vi "main(Test DQMH modules).vi"() -> ()   [LabVIEW 2018, in "Application.lvlib"] (continued)
          frame condition #1 {
          }
        }
        n847 = local read "CE14  Module did it"() -> (w1974:bool[])
        n848 = for {
          N: 6 -> [_]
          tunnel: [w2008] -> w1986 mode=indexing
          tunnel: [w2007] -> w1970 mode=indexing
          i -> [w2010]
          n849 = Increment(x=w2010) -> (x+1=w2009:i32)
          n850 = Wait (ms)(milliseconds to wait=u32 50) -> ()  [unwired: 1 out]
          n851 = call "CE14.CheckConnected.vi"("Module ID"=w2009) -> ("error out"=w2007:errorcluster, "Success"=w2008:bool)  [unwired: 8 in, 1 out]
        }
        "EMIC connected" <- w1986
        n852 = And(x=w1974, y=w1986) -> (x .and. y?=w1977:bool[])
        n853 = Index Array(array=w1977) -> (element #1=→"Inst. 4":bool, element #2=→"Inst. 5":bool, element #3=→"Inst. 6":bool, element #4=→"Inst. 7":bool, element #5=→"Inst. 8":bool, element #6=→"Inst. 9":bool)  [unwired: 6 in]
        n854 = for {
          tunnel: w1977 -> [w1999] mode=indexing
          tunnel: [w1998] -> w1976
          n855 = call "FGV Init phase.vi"("Boolean"=w1999) -> ("Init Completed?"=w1998:bool)  [unwired: 9 in, 1 out]
        }
        n856 = case shown="True" w1976 {
          tunnel: w1975 -> [_ w1997]
          tunnel: [_ w1995] -> w1972
          frame False {
          }
          frame True {
            n857 = call "App enquece.vi"("command"="INIT.Read DRV code", "queue in"=w1997) -> ("error out"=w1995:errorcluster)  [unwired: 8 in, 1 out]
          }
        }
        n858 = Merge Errors(w1971, w1970, w1972) -> (w1973:errorcluster)
        n859 = flat-sequence {
          tunnel: [w2000] -> w1979
          tunnel: w1973 -> [w2000]
          frame #0 {
            n860 = Wait (ms)(milliseconds to wait=u32 70) -> ()  [unwired: 1 out]
          }
        }
      }
      frame "MEAS.Set DMM config" {
        n861 = disable-structure shown="LOGGING==TRUE" {
          disable-tunnel: w2014 -> [w2033 _]
          frame condition #0 (active) {
            n862 = Empty String/Path?(string/path=w2033) -> (empty?=w2035:bool)
            n863 = Select(t="Quece timeout", s=w2035, f=w2033) -> (s? t:f=w2032:string)
            n864 = call "string log (SubVI).vi"("state Name"=w2032) -> ()  [unwired: 9 in, 2 out]
          }
          frame condition #1 {
          }
        }
        n865 = Variant To Data(type=T19 {"DMM config cluster"={"DCV range"=0.0, "DCI range"=0.0, "Detector Rate"=0}, "mux2-1(DMM I) encode"=enum."DMM I (0.5)"} ("DMM all config"), Variant=w2026) -> (data=w2024:T19)  [unwired: 1 in, 1 out]
        n866 = Unbundle By Name(w2024) -> ("DMM config cluster"=w2023:T20)
        n867 = Unbundle By Name(w2023) -> ("DCV range"=w2022:dbl, "DCI range"=w2021:dbl, "Detector Rate"=w2020:u8)
        n868 = call "config channel.vi"("Detector Rate"=w2020, "DCI range"=w2021, "DCV range"=w2022) -> ("error out"=w2018:errorcluster)  [unwired: 8 in]
        n869 = Merge Errors(w2015, w2018) -> (w2012:errorcluster)
        n870 = flat-sequence {
          tunnel: [w2031] -> w2013
          tunnel: w2012 -> [w2031]
          frame #0 {
            n871 = Wait (ms)(milliseconds to wait=u32 70) -> ()  [unwired: 1 out]
          }
        }
      }
      frame "MEAS.AllRelaysOFF" {
        n872 = disable-structure shown="LOGGING==TRUE" {
          disable-tunnel: w2039 -> [w2049 _]
          frame condition #0 (active) {
            n873 = Empty String/Path?(string/path=w2049) -> (empty?=w2051:bool)
            n874 = Select(t="Quece timeout", s=w2051, f=w2049) -> (s? t:f=w2048:string)
            n875 = call "string log (SubVI).vi"("state Name"=w2048) -> ()  [unwired: 9 in, 2 out]
          }
          frame condition #1 {
          }
        }
        n876 = for {
          N: 5 -> [_]
          tunnel: [w2052] -> w2044 mode=indexing
          i -> [w2054]
          n877 = case shown="5.., Default" w2054 {
            tunnel: [w2058 w2059 w2060 w2061 w2062 _] -> w2052
            frame 0 {
              n878 = Initialize Array(FALSE, 6 ("dimension size")) -> (w2055:bool[])
              n879 = call "MB01_eMICs.vi"("Array"=w2055) -> ("error out"=w2058:errorcluster)  [unwired: 10 in]
            }
            frame 1 {
              n880 = call "demux1-10_chan0.vi"() -> ("error out"=w2059:errorcluster)  [unwired: 11 in]
            }
            frame 2 {
              n881 = call "SC enable OFF.vi"() -> ("error out"=w2060:errorcluster)  [unwired: 11 in]
            }
            frame 3 {
              n882 = call "mux10-1_chan0.vi"() -> ("error out"=w2061:errorcluster)  [unwired: 11 in]
            }
            frame 4 {
              n883 = call "mux6-1_chan0.vi"() -> ("error out"=w2062:errorcluster)  [unwired: 11 in]
            }
            frame 5.., Default {
            }
          }
          n884 = Wait (ms)(milliseconds to wait=u32 70) -> ()  [unwired: 1 out]
        }
        n885 = Merge Errors(w2040, w2044) -> (w2037:errorcluster)
      }
      frame "MEAS.AllRelaysOFF2" {
        # "Turn eMICs' relays OFF"
        n886 = disable-structure shown="LOGGING==TRUE" {
          disable-tunnel: w2067 -> [w2080 _]
          frame condition #0 (active) {
            n887 = Empty String/Path?(string/path=w2080) -> (empty?=w2082:bool)
            n888 = Select(t="Quece timeout", s=w2082, f=w2080) -> (s? t:f=w2079:string)
            n889 = call "string log (SubVI).vi"("state Name"=w2079) -> ()  [unwired: 9 in, 2 out]
          }
          frame condition #1 {
          }
        }
        n890 = flat-sequence {
          tunnel: [w2078] -> w2065
          frame #0 {
            n891 = Initialize Array(FALSE, 6 ("dimension size")) -> (w2077:bool[])
            n892 = Wait (ms)(milliseconds to wait=u32 70) -> ()  [unwired: 1 out]
            n893 = call "MB01_eMICs.vi"("Array"=w2077) -> ("error out"=w2078:errorcluster)  [unwired: 10 in]
          }
        }
        n894 = Merge Errors(w2068, w2065) -> (w2064:errorcluster)
      }
      frame "MEAS.Read TRIGGER" {
        w2096 = T8 {"new board?"=TRUE, "new trigger"=TRUE, "last trigger"=TRUE}  # trigger infor
        # "JIG locked - rising-edge event"
        n895 = disable-structure shown="LOGGING==TRUE" {
          disable-tunnel: w2100 -> [w2111 _]
          frame condition #0 (active) {
            n896 = Empty String/Path?(string/path=w2111) -> (empty?=w2113:bool)
            n897 = Select(t="Quece timeout", s=w2113, f=w2111) -> (s? t:f=w2110:string)
            n898 = call "string log (SubVI).vi"("state Name"=w2110) -> ()  [unwired: 9 in, 2 out]
          }
          frame condition #1 {
          }
        }
        n899 = call "Read JIG trigger.vi"() -> ("error out"=w2083:errorcluster, "Trigger?"=w2087:bool)  [unwired: 9 in, 1 out]
        "trigger Value" <- w2087
        n900 = feedback-in #3(w2087) -> ()
        n901 = feedback #3(FALSE) -> (w2094:bool)
        n902 = Greater?(x=w2087, y=w2094) -> (0:w2089:bool)
        n903 = local read "Auto/Man"() -> (w2086:bool)
        n904 = Bundle By Name(cluster=w2096, "new board?"=w2089, "new trigger"=w2087, "last trigger"=w2094) -> (w2095:T8)
        n905 = local write "New board?"(w2089) -> ()
        n906 = local write "new Trigger?"(w2087) -> ()
        n907 = local write "last Trigger?"(w2094) -> ()
        n908 = Select(t=-1, s=w2089, f=w2091) -> (s? t:f=w2092:i32)
        n909 = And(x=w2086, y=w2089) -> (x .and. y?=w2088:bool)
        n910 = case shown="True" w2088 {
          tunnel: w2097 -> [_ w2109]
          tunnel: w2095 -> [_ w2108]
          tunnel: [_ w2107] -> w2084
          frame False {
          }
          frame True {
            n911 = Generate User Event(user event=w2109, event data cluster=w2108) -> (error out=w2107:errorcluster)  [unwired: 2 in, 1 out]
          }
        }
        n912 = Merge Errors(w2085, w2083, w2084) -> (w2098:errorcluster)
        n913 = flat-sequence {
          tunnel: [w2114] -> w2101
          tunnel: w2098 -> [w2114]
          frame #0 {
            n914 = Wait (ms)(milliseconds to wait=u32 10) -> ()  [unwired: 1 out]
          }
        }
      }
      frame "MEAS.Sel Input Current" {
        n915 = disable-structure shown="LOGGING==TRUE" {
          disable-tunnel: w2117 -> [w2132 _]
          frame condition #0 (active) {
            n916 = Empty String/Path?(string/path=w2132) -> (empty?=w2134:bool)
            n917 = Select(t="Quece timeout", s=w2134, f=w2132) -> (s? t:f=w2131:string)
            n918 = call "string log (SubVI).vi"("state Name"=w2131) -> ()  [unwired: 9 in, 2 out]
          }
          frame condition #1 {
          }
        }
        n919 = Variant To Data(type=enum16{"DMM I (0.5)", "DMM I (12)"}."DMM I (0.5)" ("mux2-1(DMM I) encode"), Variant=w2125) -> (data=w2124:enum16{"DMM I (0.5)", "DMM I (12)"})  [unwired: 1 in, 1 out]
        n920 = call "DMM I 0.5_10.vi"("mux2-1(DMM I) encode"=w2124) -> ("error out"=w2127:errorcluster)  [unwired: 10 in]
        n921 = Merge Errors(w2120, w2127) -> (w2118:errorcluster)
        n922 = flat-sequence {
          tunnel: [w2135] -> w2119
          tunnel: w2118 -> [w2135]
          frame #0 {
            n923 = Wait (ms)(milliseconds to wait=u32 70) -> ()  [unwired: 1 out]
          }
        }
      }
      frame "MEAS.Read Optos" {
        n924 = disable-structure shown="LOGGING==TRUE" {
          disable-tunnel: w2141 -> [w2165 _]
          frame condition #0 (active) {
            n925 = Empty String/Path?(string/path=w2165) -> (empty?=w2167:bool)
            n926 = Select(t="Quece timeout", s=w2167, f=w2165) -> (s? t:f=w2164:string)
            n927 = call "string log (SubVI).vi"("state Name"=w2164) -> ()  [unwired: 9 in, 2 out]
          }
          frame condition #1 {
          }
        }
        n928 = flat-sequence {
          tunnel: [w2154] -> w2139
          frame #0 {
            n929 = disable-structure shown="Enabled" {
              frame Enabled {
                n930 = Wait (ms)(milliseconds to wait=u32 100) -> ()  [unwired: 1 out]
              }
              frame Disabled {
              }
            }
            n931 = Initialize Array(FALSE, 6 ("dimension size"), 10 ("dimension size")) -> (w2149:bool[][])
            n932 = local write "Short DRV"(w2149) -> ()
          }
          frame #1 {
            n933 = call "inst.Optos.vi"() -> ("error out"=w2163:errorcluster, "Optos"=w2161:bool[])  [unwired: 9 in, 1 out]
            n934 = Reshape Array(w2161, 10 ("dimension size"), 6 ("dimension size")) -> (w2159:bool[][])
            n935 = To Variant(anything=w2161) -> (Variant=w2162:variant)
            n936 = Transpose 2D Array(2D array=w2159) -> (transposed array=→"Short DRV":bool[][])
            n937 = call "FGV Driver Data.vi"("Mode"=DUT_data_Mode."Short Circuits", "error in (no error)"=w2163, "FGV enum(Read)"=FGV_DRV_data."Write" ("FGV DRV data enum"), "data"=w2162) -> ("error out"=w2154:errorcluster)  [unwired: 4 in, 3 out]
          }
        }
        n938 = Merge Errors(w2140, w2139) -> (w2137:errorcluster)
        n939 = flat-sequence {
          tunnel: [w2168] -> w2142
          tunnel: w2137 -> [w2168]
          frame #0 {
            n940 = Wait (ms)(milliseconds to wait=u32 70) -> ()  [unwired: 1 out]
          }
        }
      }
      frame "MEAS.Reset JIG" {
        n941 = disable-structure shown="LOGGING==TRUE" {
          disable-tunnel: w2174 -> [w2185 _]
          frame condition #0 (active) {
            n942 = Empty String/Path?(string/path=w2185) -> (empty?=w2187:bool)
            n943 = Select(t="Quece timeout", s=w2187, f=w2185) -> (s? t:f=w2184:string)
            n944 = call "string log (SubVI).vi"("state Name"=w2184) -> ()  [unwired: 9 in, 2 out]
          }
          frame condition #1 {
          }
        }
        n945 = call "JIG Reset.vi"() -> ("error out"=w2179:errorcluster)  [unwired: 11 in]
        n946 = Merge Errors(w2175, w2179) -> (w2170:errorcluster)
        n947 = flat-sequence {
          tunnel: [w2182] -> w2171
          tunnel: w2170 -> [w2182]
          frame #0 {
            n948 = Wait (ms)(milliseconds to wait=u32 100) -> ()  [unwired: 1 out]
          }
        }
      }
      frame "MEAS.Turn+5V" {
        n949 = disable-structure shown="LOGGING==TRUE" {
          disable-tunnel: w2190 -> [w2206 _]
          frame condition #0 (active) {
            n950 = Empty String/Path?(string/path=w2206) -> (empty?=w2208:bool)
            n951 = Select(t="Quece timeout", s=w2208, f=w2206) -> (s? t:f=w2205:string)
            n952 = call "string log (SubVI).vi"("state Name"=w2205) -> ()  [unwired: 9 in, 2 out]
          }
          frame condition #1 {
          }
        }
        n953 = Variant To Data(type=TRUE, Variant=w2199) -> (data=w2189:bool)  [unwired: 1 in, 1 out]
        n954 = case shown="False" w2189 {
          tunnel: [w2203 w2204] -> w2196
          frame False {
            n955 = call "SC enable OFF.vi"() -> ("error out"=w2203:errorcluster)  [unwired: 11 in]
          }
          frame True {
            n956 = call "SC enable ON.vi"() -> ("error out"=w2204:errorcluster)  [unwired: 11 in]
          }
        }
        n957 = Merge Errors(w2191, w2196) -> (w2192:errorcluster)
        n958 = flat-sequence {
          tunnel: w2192 -> [w2209]
          tunnel: [w2209] -> w2195
          frame #0 {
            n959 = Wait (ms)(milliseconds to wait=u32 2000) -> ()  [unwired: 1 out]
          }
        }
      }
      frame "MEAS.demux1-10" {
        n960 = disable-structure shown="LOGGING==TRUE" {
          disable-tunnel: w2214 -> [w2240 _]
          frame condition #0 (active) {
            n961 = Empty String/Path?(string/path=w2240) -> (empty?=w2242:bool)
            n962 = Select(t="Quece timeout", s=w2242, f=w2240) -> (s? t:f=w2239:string)
            n963 = call "string log (SubVI).vi"("state Name"=w2239) -> ()  [unwired: 9 in, 2 out]
          }
          frame condition #1 {
          }
        }
        n964 = Variant To Data(type=T4."demux1_10_channel0" ("demux1_10(x6)_encode"), Variant=w2222) -> (data=w2213:T4)  [unwired: 1 in, 1 out]
        n965 = case shown="\"demux1_10_channel7\"" w2213 {
          tunnel: [w2228 w2229 w2230 w2231 w2232 w2233 w2234 w2235 w2236 w2237 w2238] -> w2212
          frame "demux1_10_channel0", Default {
            n966 = call "demux1-10_chan0.vi"() -> ("error out"=w2228:errorcluster)  [unwired: 11 in]
          }
          frame "demux1_10_channel1" {
            n967 = call "demux1-10_chan1.vi"() -> ("error out"=w2229:errorcluster)  [unwired: 11 in]
          }
          frame "demux1_10_channel2" {
            n968 = call "demux1-10_chan2.vi"() -> ("error out"=w2230:errorcluster)  [unwired: 11 in]
          }
          frame "demux1_10_channel3" {
            n969 = call "demux1-10_chan3.vi"() -> ("error out"=w2231:errorcluster)  [unwired: 11 in]
          }
          frame "demux1_10_channel4" {
            n970 = call "demux1-10_chan4.vi"() -> ("error out"=w2232:errorcluster)  [unwired: 11 in]
          }
          frame "demux1_10_channel5" {
            n971 = call "demux1-10_chan5.vi"() -> ("error out"=w2233:errorcluster)  [unwired: 11 in]
          }
          frame "demux1_10_channel6" {
            n972 = call "demux1-10_chan6.vi"() -> ("error out"=w2234:errorcluster)  [unwired: 11 in]
          }
          frame "demux1_10_channel7" {
            n973 = call "demux1-10_chan7.vi"() -> ("error out"=w2235:errorcluster)  [unwired: 11 in]
          }
          frame "demux1_10_channel8" {
            n974 = call "demux1-10_chan8.vi"() -> ("error out"=w2236:errorcluster)  [unwired: 11 in]
          }
          frame "demux1_10_channel9" {
            n975 = call "demux1-10_chan9.vi"() -> ("error out"=w2237:errorcluster)  [unwired: 11 in]
          }
          frame "demux1_10_channel10" {
            n976 = call "demux1-10_chan10.vi"() -> ("error out"=w2238:errorcluster)  [unwired: 11 in]
          }
        }
        n977 = Merge Errors(w2215, w2212) -> (w2216:errorcluster)
        n978 = flat-sequence {
          tunnel: [w2226] -> w2217
          tunnel: w2216 -> [w2226]
          frame #0 {
            n979 = Wait (ms)(milliseconds to wait=u32 100 ("1-10delay")) -> ()  [unwired: 1 out]
          }
        }
      }
      frame "MEAS.eMIC" {
        # "eliminated shorted Circuits"
        n980 = disable-structure shown="LOGGING==TRUE" {
          disable-tunnel: w2245 -> [w2267 _]
          frame condition #0 (active) {
            n981 = Empty String/Path?(string/path=w2267) -> (empty?=w2269:bool)
            n982 = Select(t="Quece timeout", s=w2269, f=w2267) -> (s? t:f=w2266:string)
            n983 = call "string log (SubVI).vi"("state Name"=w2266) -> ()  [unwired: 9 in, 2 out]
          }
          frame condition #1 {
          }
        }
        n984 = Variant To Data(type=bool[] [], Variant=w2260) -> (data=w2254:bool[])  [unwired: 1 in, 1 out]
        n985 = call "FGV Driver Data.vi"("DUT channel (1-11)"=w2247) -> ("Short Circuits?"=w2256:bool[])  [unwired: 7 in, 3 out]
        n986 = Not(x=w2256) -> (.not. x?=w2255:bool[])
        n987 = And(x=w2255, y=w2254) -> (x .and. y?=w2253:bool[])
        n988 = call "MB01_eMICs.vi"("Array"=w2253) -> ("error out"=w2251:errorcluster)  [unwired: 10 in]
        n989 = call "FGV wait for 6 eMICs.vi"("Enum"=enum16{"Init", "count"}."Init", "error in (no error)"=w2251) -> ("error out"=w2243:errorcluster, "wait done"=w2252:bool)  [unwired: 7 in, 1 out]
        n990 = local write "AC  Completed"(w2252) -> ()
        n991 = Merge Errors(w2246, w2243) -> (w2248:errorcluster)
        n992 = flat-sequence {
          tunnel: [w2265] -> w2249
          tunnel: w2248 -> [w2265]
          frame #0 {
            n993 = Wait (ms)(milliseconds to wait=u32 100 ("eMIC delay")) -> ()  [unwired: 1 out]
          }
        }
      }
      frame "MEAS.requestAC" {
        n994 = disable-structure shown="LOGGING==TRUE" {
          disable-tunnel: w2273 -> [w2296 _]
          frame condition #0 (active) {
            n995 = Empty String/Path?(string/path=w2296) -> (empty?=w2298:bool)
            n996 = Select(t="Quece timeout", s=w2298, f=w2296) -> (s? t:f=w2295:string)
            n997 = call "string log (SubVI).vi"("state Name"=w2295) -> ()  [unwired: 9 in, 2 out]
          }
          frame condition #1 {
          }
        }
        n998 = Variant To Data(type=-1 ("Module ID"), Variant=w2271) -> (data=w2270:i32)  [unwired: 1 in, 1 out]
        n999 = case shown="1, Default" w2270 {
          selector: w2270 -> [w2289 _]
          tunnel: [w2288 w2293] -> w2276
          frame 1, Default {
            n1000 = Quotient & Remainder(x=w2289, y=6) -> (x-y*floor(x/y)=w2285:i32)  [unwired: 1 out]
            n1001 = Equal To 0?(x=w2285) -> (x = 0?=w2287:bool)
            n1002 = Select(t=6, s=w2287, f=w2285) -> (s? t:f=w2284:i32)
            n1003 = call "Read AC parameters.vi"("Module ID"=w2284) -> ("error out"=w2288:errorcluster)  [unwired: 10 in]
          }
          frame 0 {
            n1004 = call "FGV wait for 6 eMICs.vi"("Enum"=enum16{"Init", "count"}."Init") -> ("error out"=w2291:errorcluster)  [unwired: 8 in, 2 out]
            n1005 = call "Read AC parameters.vi"("error in"=w2291, "Module ID"=-1) -> ("error out"=w2293:errorcluster)  [unwired: 9 in]
          }
        }
        n1006 = Merge Errors(w2277, w2276) -> (w2275:errorcluster)
      }
      frame "MEAS.mux6_1" {
        n1007 = disable-structure shown="LOGGING==TRUE" {
          disable-tunnel: w2306 -> [w2343 _]
          frame condition #0 (active) {
            n1008 = Empty String/Path?(string/path=w2343) -> (empty?=w2345:bool)
            n1009 = Select(t="Quece timeout", s=w2345, f=w2343) -> (s? t:f=w2342:string)
            n1010 = call "string log (SubVI).vi"("state Name"=w2342) -> ()  [unwired: 9 in, 2 out]
          }
          frame condition #1 {
          }
        }
        n1011 = Variant To Data(type=T2."mux6-1_channel0" ("mux6_1(3wires)_encode"), Variant=w2312) -> (data=w2305:T2)  [unwired: 1 in, 1 out]
        n1012 = case shown="\"mux6_1_channel1_3\"" w2305 {
          tunnel: [w2317 w2319 w2321 w2323 w2325 w2327 w2329 w2331 w2333 w2335 w2337 w2339 w2341] -> w2304
          tunnel: [w2316 w2318 w2320 w2322 w2324 w2326 w2328 w2330 w2332 w2334 w2336 w2338 w2340] -> w2300
          tunnel: u32 180 ("6_1 delay") -> [w2316 _ w2320 _ w2324 _ w2328 _ w2332 _ w2336 _ w2340]
          tunnel: u32 70 ("6_1 delay2") -> [_ w2318 _ w2322 _ w2326 _ w2330 _ w2334 _ w2338 _]
          frame "mux6-1_channel0", Default {
            n1013 = call "mux6-1_chan0.vi"() -> ("error out"=w2317:errorcluster)  [unwired: 11 in]
          }
          frame "mux6-1_channel1_2" {
            n1014 = call "mux6-1_chan1_1.vi"() -> ("error out"=w2319:errorcluster)  [unwired: 11 in]
          }
          frame "mux6_1_channel1_3" {
            n1015 = call "mux6-1_chan1_2.vi"() -> ("error out"=w2321:errorcluster)  [unwired: 11 in]
          }
          frame "mux6_1_channel2_2" {
            n1016 = call "mux6-1_chan2_1.vi"() -> ("error out"=w2323:errorcluster)  [unwired: 11 in]
          }
          frame "mux6_1_channel2_3" {
            n1017 = call "mux6-1_chan2_2.vi"() -> ("error out"=w2325:errorcluster)  [unwired: 11 in]
          }
          frame "mux6_1_channel3_2" {
            n1018 = call "mux6-1_chan3_1.vi"() -> ("error out"=w2327:errorcluster)  [unwired: 11 in]
          }
          frame "mux6_1_channel3_3" {
            n1019 = call "mux6-1_chan3_2.vi"() -> ("error out"=w2329:errorcluster)  [unwired: 11 in]
          }
          frame "mux6_1_channel4_2" {
            n1020 = call "mux6-1_chan4_1.vi"() -> ("error out"=w2331:errorcluster)  [unwired: 11 in]
          }
          frame "mux6_1_channel4_3" {
            n1021 = call "mux6-1_chan4_2.vi"() -> ("error out"=w2333:errorcluster)  [unwired: 11 in]
          }
          frame "mux6_1_channel5_2" {
            n1022 = call "mux6-1_chan5_1.vi"() -> ("error out"=w2335:errorcluster)  [unwired: 11 in]
          }
          frame "mux6_1_channel5_3" {
            n1023 = call "mux6-1_chan5_2.vi"() -> ("error out"=w2337:errorcluster)  [unwired: 11 in]
          }
          frame "mux6_1_channel6_2" {
            n1024 = call "mux6-1_chan6_1.vi"() -> ("error out"=w2339:errorcluster)  [unwired: 11 in]
          }
          frame "mux6_1_channel6_3" {
            n1025 = call "mux6-1_chan6_2.vi"() -> ("error out"=w2341:errorcluster)  [unwired: 11 in]
          }
        }
        n1026 = Wait (ms)(milliseconds to wait=w2300) -> ()  [unwired: 1 out]
        n1027 = Merge Errors(w2307, w2304) -> (w2299:errorcluster)
      }
      frame "MEAS.mux10-1" {
        n1028 = disable-structure shown="LOGGING==TRUE" {
          disable-tunnel: w2349 -> [w2375 _]
          frame condition #0 (active) {
            n1029 = Empty String/Path?(string/path=w2375) -> (empty?=w2377:bool)
            n1030 = Select(t="Quece timeout", s=w2377, f=w2375) -> (s? t:f=w2374:string)
            n1031 = call "string log (SubVI).vi"("state Name"=w2374) -> ()  [unwired: 9 in, 2 out]
          }
          frame condition #1 {
          }
        }
        n1032 = Variant To Data(type=T3."mux10_1_channel0" ("mux10_1(x6)_encode"), Variant=w2357) -> (data=w2348:T3)  [unwired: 1 in, 1 out]
        n1033 = case shown="\"mux10_1_channel10\"" w2348 {
          tunnel: [w2363 w2364 w2365 w2366 w2367 w2368 w2369 w2370 w2371 w2372 w2373] -> w2347
          frame "mux10_1_channel0", Default {
            n1034 = call "mux10-1_chan0.vi"() -> ("error out"=w2363:errorcluster)  [unwired: 11 in]
          }
          frame "mux10_1_channel1" {
            n1035 = call "mux10-1_chan1.vi"() -> ("error out"=w2364:errorcluster)  [unwired: 11 in]
          }
          frame "mux10_1_channel2" {
            n1036 = call "mux10-1_chan2.vi"() -> ("error out"=w2365:errorcluster)  [unwired: 11 in]
          }
          frame "mux10_1_channel3" {
            n1037 = call "mux10-1_chan3.vi"() -> ("error out"=w2366:errorcluster)  [unwired: 11 in]
          }
          frame "mux10_1_channel4" {
            n1038 = call "mux10-1_chan4.vi"() -> ("error out"=w2367:errorcluster)  [unwired: 11 in]
          }
          frame "mux10_1_channel5" {
            n1039 = call "mux10-1_chan5.vi"() -> ("error out"=w2368:errorcluster)  [unwired: 11 in]
          }
          frame "mux10_1_channel6" {
            n1040 = call "mux10-1_chan6.vi"() -> ("error out"=w2369:errorcluster)  [unwired: 11 in]
          }
          frame "mux10_1_channel7" {
            n1041 = call "mux10-1_chan7.vi"() -> ("error out"=w2370:errorcluster)  [unwired: 11 in]
          }
          frame "mux10_1_channel8" {
            n1042 = call "mux10-1_chan8.vi"() -> ("error out"=w2371:errorcluster)  [unwired: 11 in]
          }
          frame "mux10_1_channel9" {
            n1043 = call "mux10-1_chan9.vi"() -> ("error out"=w2372:errorcluster)  [unwired: 11 in]
          }
          frame "mux10_1_channel10" {
            n1044 = call "mux10-1_chan10.vi"() -> ("error out"=w2373:errorcluster)  [unwired: 11 in]
          }
        }
        n1045 = Merge Errors(w2352, w2347) -> (w2351:errorcluster)
        n1046 = flat-sequence {
          tunnel: w2351 -> [w2361]
          tunnel: [w2361] -> w2350
          frame #0 {
            n1047 = Wait (ms)(milliseconds to wait=u32 100 ("10-1 delay")) -> ()  [unwired: 1 out]
          }
        }
      }
      frame "MEAS.DMM dual read" {
        n1048 = disable-structure shown="LOGGING==TRUE" {
          disable-tunnel: w2385 -> [w2410 _]
          frame condition #0 (active) {
            n1049 = Empty String/Path?(string/path=w2410) -> (empty?=w2413:bool)
            n1050 = Select(t="Quece timeout", s=w2413, f=w2410) -> (s? t:f=w2411:string)
            n1051 = call "string log (SubVI).vi"("state Name"=w2411) -> ()  [unwired: 9 in, 2 out]
          }
          frame condition #1 {
          }
        }
        n1052 = call "FGV Driver Data.vi"("DUT index(1-60)"=w2378) -> ("DUT SC"=w2379:bool)  [unwired: 7 in, 3 out]
        n1053 = case shown="True" w2379 {
          tunnel: [w2392 _] -> w2381
          tunnel: w2378 -> [w2393 _]
          frame False {
            n1054 = flat-sequence {
              tunnel: [w2396] -> w2394
              tunnel: w2393 -> [w2396]
              tunnel: w2394 -> [w2399]
              tunnel: [w2398] -> w2392
              frame #0 {
                w2395 = 0.0 ("DCV(Volts)")
                n1055 = disable-structure shown="Enabled" {
                  frame Enabled {
                    n1056 = Wait (ms)(milliseconds to wait=u32 50) -> ()  [unwired: 1 out]
                  }
                  frame Disabled {
                  }
                }
                n1057 = local write "DCV(Volts)"(w2395) -> ()
                n1058 = local write "DCI(mA)"(w2395) -> ()
              }
              frame #1 {
                w2400 = u16 2 items=["1st Display", "2nd Display", "1st & 2nd Display"] ("Sets to Display")
                n1059 = call "Read DCV_DCI.vi"("Sets to Display"=w2400) -> ("error out"=w2403:errorcluster, "DCI"=w2407:dbl, "DCV"=w2406:dbl)  [unwired: 7 in, 1 out]
                "DCI(mA)" <- w2407
                "DCV(Volts)" <- w2406
                n1060 = Build Array(w2406, w2407) -> (w2405:dbl[])
                n1061 = To Variant(anything=w2405) -> (Variant=w2404:variant)
                n1062 = call "FGV Driver Data.vi"("Mode"=DUT_data_Mode."DC parameter", "DUT index(1-60)"=w2399, "error in (no error)"=w2403, "FGV enum(Read)"=FGV_DRV_data."Write" ("FGV DRV data enum"), "data"=w2404) -> ("error out"=w2398:errorcluster)  [unwired: 3 in, 3 out]
              }
            }
          }
          frame True {
          }
        }
        n1063 = Merge Errors(w2386, w2381) -> (w2383:errorcluster)
        n1064 = flat-sequence {
          tunnel: [w2409] -> w2384
          tunnel: w2383 -> [w2409]
          frame #0 {
            n1065 = Wait (ms)(milliseconds to wait=u32 10 ("DMM delay")) -> ()  [unwired: 1 out]
          }
        }
      }
      frame "Test Shorted Circuits" {
        w2422 = T24 {"command"="", "Data"=variant} ("Variant")
        n1066 = disable-structure shown="LOGGING==TRUE" {
          disable-tunnel: w2428 -> [w2448 _]
          frame condition #0 (active) {
            n1067 = Empty String/Path?(string/path=w2448) -> (empty?=w2450:bool)
            n1068 = Select(t="Quece timeout", s=w2450, f=w2448) -> (s? t:f=w2447:string)
            n1069 = call "string log (SubVI).vi"("state Name"=w2447) -> ()  [unwired: 9 in, 2 out]
          }
          frame condition #1 {
          }
        }
        n1070 = To Variant(anything=TRUE) -> (Variant=w2438:variant)
        n1071 = To Variant(anything=FALSE) -> (Variant=w2424:variant)
        n1072 = Bundle By Name(cluster=w2422, "command"="MEAS.AllRelaysOFF") -> (w2440:T24)
        n1073 = Bundle By Name(cluster=w2422, "command"="MEAS.Turn+5V", "Data"=w2438) -> (w2439:T24)
        n1074 = Bundle By Name(cluster=w2422, "command"="MEAS.Read Optos") -> (w2436:T24)
        n1075 = Bundle By Name(cluster=w2422, "command"="MEAS.Turn+5V", "Data"=w2424) -> (w2427:T24)
        n1076 = Bundle By Name(cluster=w2422, "command"="Apps.UI Update SC") -> (w2420:T24)
        n1077 = Build Array(w2440, w2439, w2436, w2427, w2420) -> (w2429:T24[])
        n1078 = Reverse 1D Array(array=w2429) -> (reversed array=w2430:T24[])
        n1079 = for {
          tunnel: w2430 -> [w2454] mode=indexing
          tunnel: w2434 -> [w2456]
          tunnel: [w2455] -> w2414 mode=indexing
          n1080 = Unbundle By Name(w2454) -> ("command"=w2453:string, "Data"=w2452:variant)
          n1081 = call "App enquece.vi"("Priority Enquece"=TRUE, "command data"=w2452, "command"=w2453, "queue in"=w2456) -> ("error out"=w2455:errorcluster)  [unwired: 6 in, 1 out]
        }
        n1082 = call "reset DRV UI (SubVI).vi"("Ref  in"=w2433) -> ("error out"=w2417:errorcluster)  [unwired: 9 in, 1 out]
        n1083 = call "FGV Driver Data.vi"("error in (no error)"=w2417, "FGV enum(Read)"=FGV_DRV_data."Init" ("FGV DRV data enum")) -> ("error out"=w2415:errorcluster)  [unwired: 6 in, 3 out]
        n1084 = Merge Errors(w2416, w2415, w2414) -> (w2419:errorcluster)
      }
      frame "Test Channel 1" {
        w2463 = T9 {"command"="", "data"=variant} ("element")
        w2497 = 1  # DUT channel (1-11)
        n1085 = disable-structure shown="LOGGING==TRUE" {
          disable-tunnel: w2493 -> [w2523 _]
          frame condition #0 (active) {
            n1086 = Empty String/Path?(string/path=w2523) -> (empty?=w2525:bool)
            n1087 = Select(t="Quece timeout", s=w2525, f=w2523) -> (s? t:f=w2522:string)
            n1088 = call "string log (SubVI).vi"("state Name"=w2522) -> ()  [unwired: 9 in, 2 out]
          }
          frame condition #1 {
          }
        }
        n1089 = Build Array("Apps.WaitForEvent", "MEAS.AllRelaysOFF2", "Apps.UI Update") -> (w2459:string[])
        n1090 = Reverse 1D Array(array=w2459) -> (reversed array=w2458:string[])
        n1091 = for {
          tunnel: [w2513] -> w2483 mode=indexing
          shift-right: [w2512] -> w2482
          shift-left: w2484 -> [w2515]
          tunnel: w2458 -> [w2511] mode=indexing
          n1092 = call "App enquece.vi"("Priority Enquece"=TRUE, "command"=w2511, "queue in"=w2515) -> ("error out"=w2513:errorcluster, "Queue out"=w2512:refnum<queue>)  [unwired: 7 in]
        }
        n1093 = call "FGV DRV stand.vi"() -> ("Sub-Test.DCV"=w2477:bool)  [unwired: 10 in, 1 out]
        n1094 = Merge Errors(w2483) -> (w2480:errorcluster)
        n1095 = case shown="False" w2477 {
          tunnel: [w2500 w2510] -> w2490
          frame False {
            n1096 = Build Array("WaitFor", "MEAS.requestAC") -> (w2500:string[])
          }
          frame True {
            n1097 = Build Array("Test DRV 1", "Test DRV 2", "Test DRV 3", "Test DRV 4", "Test DRV 5", "Test DRV 6", "MEAS.requestAC") -> (w2510:string[])
          }
        }
        n1098 = Reverse 1D Array(array=w2490) -> (reversed array=w2491:string[])
        n1099 = for {
          tunnel: w2491 -> [w2520] mode=indexing
          tunnel: [w2519] -> w2488 mode=indexing
          shift-right: [w2518] -> w2489
          shift-left: w2482 -> [w2521]
          tunnel: w2480 -> [w2517]
          n1100 = call "App enquece.vi"("Priority Enquece"=TRUE, "error in (no error)"=w2517, "command"=w2520, "queue in"=w2521) -> ("error out"=w2519:errorcluster, "Queue out"=w2518:refnum<queue>)  [unwired: 6 in]
        }
        n1101 = Merge Errors(w2488) -> (w2487:errorcluster)
        n1102 = Initialize Array(TRUE, 6 ("dimension size")) -> (w2465:bool[])
        n1103 = To Variant(anything=T3."mux10_1_channel1" ("mux10_1(x6)_encode")) -> (Variant=w2475:variant)
        n1104 = To Variant(anything=T4."demux1_10_channel1" ("demux1_10(x6)_encode")) -> (Variant=w2471:variant)
        n1105 = To Variant(anything=w2465) -> (Variant=w2464:variant)
        n1106 = Bundle By Name(cluster=w2463, "command"="MEAS.mux10-1", "data"=w2475) -> (w2470:T9)
        n1107 = Bundle By Name(cluster=w2463, "command"="MEAS.demux1-10", "data"=w2471) -> (w2469:T9)
        n1108 = Bundle By Name(cluster=w2463, "command"="MEAS.eMIC", "data"=w2464) -> (w2457:T9)
        n1109 = Build Array(w2470, w2469, w2457, w2457) -> (w2486:T9[])
        n1110 = Reverse 1D Array(array=w2486) -> (reversed array=w2485:T9[])
        n1111 = for {
          tunnel: w2485 -> [w2531] mode=indexing
          tunnel: [w2528] -> w2492 mode=indexing
          tunnel: w2487 -> [w2527]
          tunnel: w2489 -> [w2532]
          n1112 = Unbundle By Name(w2531) -> ("command"=w2530:string, "data"=w2529:variant)
          n1113 = call "App enquece.vi"("Priority Enquece"=TRUE, "error in (no error)"=w2527, "command data"=w2529, "command"=w2530, "queue in"=w2532) -> ("error out"=w2528:errorcluster)  [unwired: 5 in, 1 out]
        }
        n1114 = Merge Errors(w2495, w2492) -> (w2496:errorcluster)
      }
      frame "Test Channel 2" {
        w2539 = T9 {"command"="", "data"=variant} ("element")
        w2573 = 2  # DUT channel (1-11)
        n1115 = disable-structure shown="LOGGING==TRUE" {
          disable-tunnel: w2568 -> [w2599 _]
          frame condition #0 (active) {
            n1116 = Empty String/Path?(string/path=w2599) -> (empty?=w2601:bool)
            n1117 = Select(t="Quece timeout", s=w2601, f=w2599) -> (s? t:f=w2598:string)
            n1118 = call "string log (SubVI).vi"("state Name"=w2598) -> ()  [unwired: 9 in, 2 out]
          }
          frame condition #1 {
          }
        }
        n1119 = Build Array("Apps.WaitForEvent", "MEAS.AllRelaysOFF2", "Apps.UI Update") -> (w2536:string[])
        n1120 = Reverse 1D Array(array=w2536) -> (reversed array=w2535:string[])
        n1121 = for {
          tunnel: [w2590] -> w2562 mode=indexing
          shift-right: [w2591] -> w2564
          shift-left: w2557 -> [w2589]
          tunnel: w2535 -> [w2587] mode=indexing
          n1122 = call "App enquece.vi"("Priority Enquece"=TRUE, "command"=w2587, "queue in"=w2589) -> ("error out"=w2590:errorcluster, "Queue out"=w2591:refnum<queue>)  [unwired: 7 in]
        }
        n1123 = call "FGV DRV stand.vi"() -> ("Sub-Test.DCV"=w2552:bool)  [unwired: 10 in, 1 out]
        n1124 = case shown="True" w2552 {
          tunnel: [w2576 w2586] -> w2565
          frame False {
            n1125 = Build Array("WaitFor", "MEAS.requestAC") -> (w2576:string[])
          }
          frame True {
            n1126 = Build Array("Test DRV 7", "Test DRV 8", "Test DRV 9", "Test DRV 10", "Test DRV 11", "Test DRV 12", "MEAS.requestAC") -> (w2586:string[])
          }
        }
        n1127 = Merge Errors(w2562) -> (w2556:errorcluster)
        n1128 = Reverse 1D Array(array=w2565) -> (reversed array=w2566:string[])
        n1129 = for {
          tunnel: w2566 -> [w2592] mode=indexing
          tunnel: [w2596] -> w2561 mode=indexing
          shift-right: [w2595] -> w2563
          shift-left: w2564 -> [w2597]
          tunnel: w2556 -> [w2594]
          n1130 = call "App enquece.vi"("Priority Enquece"=TRUE, "error in (no error)"=w2594, "command"=w2592, "queue in"=w2597) -> ("error out"=w2596:errorcluster, "Queue out"=w2595:refnum<queue>)  [unwired: 6 in]
        }
        n1131 = Merge Errors(w2561) -> (w2560:errorcluster)
        n1132 = Initialize Array(TRUE, 6 ("dimension size")) -> (w2542:bool[])
        n1133 = To Variant(anything=T3."mux10_1_channel2" ("mux10_1(x6)_encode")) -> (Variant=w2550:variant)
        n1134 = To Variant(anything=T4."demux1_10_channel2" ("demux1_10(x6)_encode")) -> (Variant=w2547:variant)
        n1135 = To Variant(anything=w2542) -> (Variant=w2541:variant)
        n1136 = Bundle By Name(cluster=w2539, "command"="MEAS.mux10-1", "data"=w2550) -> (w2546:T9)
        n1137 = Bundle By Name(cluster=w2539, "command"="MEAS.demux1-10", "data"=w2547) -> (w2545:T9)
        n1138 = Bundle By Name(cluster=w2539, "command"="MEAS.eMIC", "data"=w2541) -> (w2540:T9)
        n1139 = Build Array(w2546, w2545, w2540) -> (w2559:T9[])
        n1140 = Reverse 1D Array(array=w2559) -> (reversed array=w2558:T9[])
        n1141 = for {
          tunnel: w2558 -> [w2607] mode=indexing
          tunnel: [w2604] -> w2567 mode=indexing
          tunnel: w2560 -> [w2603]
          tunnel: w2563 -> [w2608]
          n1142 = Unbundle By Name(w2607) -> ("command"=w2606:string, "data"=w2605:variant)
          n1143 = call "App enquece.vi"("Priority Enquece"=TRUE, "error in (no error)"=w2603, "command data"=w2605, "command"=w2606, "queue in"=w2608) -> ("error out"=w2604:errorcluster)  [unwired: 5 in, 1 out]
        }
        n1144 = Merge Errors(w2570, w2567) -> (w2571:errorcluster)
      }
      frame "Test Channel 3" {
        w2612 = T9 {"command"="", "data"=variant} ("element")
        w2648 = 3  # DUT channel (1-11)
        n1145 = disable-structure shown="LOGGING==TRUE" {
          disable-tunnel: w2644 -> [w2674 _]
          frame condition #0 (active) {
            n1146 = Empty String/Path?(string/path=w2674) -> (empty?=w2676:bool)
            n1147 = Select(t="Quece timeout", s=w2676, f=w2674) -> (s? t:f=w2673:string)
            n1148 = call "string log (SubVI).vi"("state Name"=w2673) -> ()  [unwired: 9 in, 2 out]
          }
          frame condition #1 {
          }
        }
        n1149 = Build Array("Apps.UI Update", "MEAS.AllRelaysOFF2", "Apps.WaitForEvent") -> (w2632:string[])
        n1150 = for {
          tunnel: [w2664] -> w2638 mode=indexing
          shift-right: [w2665] -> w2640
          shift-left: w2634 -> [w2663]
          tunnel: w2632 -> [w2662] mode=indexing
          n1151 = call "App enquece.vi"("Priority Enquece"=TRUE, "command"=w2662, "queue in"=w2663) -> ("error out"=w2664:errorcluster, "Queue out"=w2665:refnum<queue>)  [unwired: 7 in]
        }
        n1152 = call "FGV DRV stand.vi"() -> ("Sub-Test.DCV"=w2626:bool)  [unwired: 10 in, 1 out]
        n1153 = Merge Errors(w2638) -> (w2610:errorcluster)
        n1154 = case shown="True" w2626 {
          tunnel: [w2651 w2661] -> w2641
          frame False {
            n1155 = Build Array("WaitFor", "MEAS.requestAC") -> (w2651:string[])
          }
          frame True {
            n1156 = Build Array("Test DRV 13", "Test DRV 14", "Test DRV 15", "Test DRV 16", "Test DRV 17", "Test DRV 18", "MEAS.requestAC") -> (w2661:string[])
          }
        }
        n1157 = Reverse 1D Array(array=w2641) -> (reversed array=w2642:string[])
        n1158 = for {
          tunnel: w2642 -> [w2671] mode=indexing
          tunnel: [w2670] -> w2628 mode=indexing
          shift-right: [w2669] -> w2639
          shift-left: w2640 -> [w2672]
          tunnel: w2610 -> [w2668]
          n1159 = call "App enquece.vi"("Priority Enquece"=TRUE, "error in (no error)"=w2668, "command"=w2671, "queue in"=w2672) -> ("error out"=w2670:errorcluster, "Queue out"=w2669:refnum<queue>)  [unwired: 6 in]
        }
        n1160 = Merge Errors(w2628) -> (w2637:errorcluster)
        n1161 = Initialize Array(TRUE, 6 ("dimension size")) -> (w2615:bool[])
        n1162 = To Variant(anything=T3."mux10_1_channel3" ("mux10_1(x6)_encode")) -> (Variant=w2624:variant)
        n1163 = To Variant(anything=T4."demux1_10_channel3" ("demux1_10(x6)_encode")) -> (Variant=w2620:variant)
        n1164 = To Variant(anything=w2615) -> (Variant=w2614:variant)
        n1165 = Bundle By Name(cluster=w2612, "command"="MEAS.mux10-1", "data"=w2624) -> (w2619:T9)
        n1166 = Bundle By Name(cluster=w2612, "command"="MEAS.demux1-10", "data"=w2620) -> (w2618:T9)
        n1167 = Bundle By Name(cluster=w2612, "command"="MEAS.eMIC", "data"=w2614) -> (w2613:T9)
        n1168 = Build Array(w2619, w2618, w2613) -> (w2636:T9[])
        n1169 = Reverse 1D Array(array=w2636) -> (reversed array=w2635:T9[])
        n1170 = for {
          tunnel: w2635 -> [w2682] mode=indexing
          tunnel: [w2679] -> w2643 mode=indexing
          tunnel: w2637 -> [w2678]
          tunnel: w2639 -> [w2683]
          n1171 = Unbundle By Name(w2682) -> ("command"=w2681:string, "data"=w2680:variant)
          n1172 = call "App enquece.vi"("Priority Enquece"=TRUE, "error in (no error)"=w2678, "command data"=w2680, "command"=w2681, "queue in"=w2683) -> ("error out"=w2679:errorcluster)  [unwired: 5 in, 1 out]
        }
        n1173 = Merge Errors(w2609, w2643) -> (w2646:errorcluster)
      }
      frame "Test Channel 4" {
        w2685 = T9 {"command"="", "data"=variant} ("element")
        w2723 = 4  # DUT channel (1-11)
        n1174 = disable-structure shown="LOGGING==TRUE" {
          disable-tunnel: w2718 -> [w2749 _]
          frame condition #0 (active) {
            n1175 = Empty String/Path?(string/path=w2749) -> (empty?=w2751:bool)
            n1176 = Select(t="Quece timeout", s=w2751, f=w2749) -> (s? t:f=w2748:string)
            n1177 = call "string log (SubVI).vi"("state Name"=w2748) -> ()  [unwired: 9 in, 2 out]
          }
          frame condition #1 {
          }
        }
        n1178 = Build Array("Apps.UI Update", "MEAS.AllRelaysOFF2", "Apps.WaitForEvent") -> (w2705:string[])
        n1179 = for {
          tunnel: [w2739] -> w2712 mode=indexing
          shift-right: [w2740] -> w2714
          shift-left: w2707 -> [w2738]
          tunnel: w2705 -> [w2737] mode=indexing
          n1180 = call "App enquece.vi"("Priority Enquece"=TRUE, "command"=w2737, "queue in"=w2738) -> ("error out"=w2739:errorcluster, "Queue out"=w2740:refnum<queue>)  [unwired: 7 in]
        }
        n1181 = Merge Errors(w2712) -> (w2704:errorcluster)
        n1182 = call "FGV DRV stand.vi"() -> ("Sub-Test.DCV"=w2700:bool)  [unwired: 10 in, 1 out]
        n1183 = case shown="True" w2700 {
          tunnel: [w2726 w2736] -> w2715
          frame False {
            n1184 = Build Array("WaitFor", "MEAS.requestAC") -> (w2726:string[])
          }
          frame True {
            n1185 = Build Array("Test DRV 19", "Test DRV 20", "Test DRV 21", "Test DRV 22", "Test DRV 23", "Test DRV 24", "MEAS.requestAC") -> (w2736:string[])
          }
        }
        n1186 = Reverse 1D Array(array=w2715) -> (reversed array=w2716:string[])
        n1187 = for {
          tunnel: w2716 -> [w2746] mode=indexing
          tunnel: [w2745] -> w2711 mode=indexing
          shift-right: [w2744] -> w2713
          shift-left: w2714 -> [w2747]
          tunnel: w2704 -> [w2743]
          n1188 = call "App enquece.vi"("Priority Enquece"=TRUE, "error in (no error)"=w2743, "command"=w2746, "queue in"=w2747) -> ("error out"=w2745:errorcluster, "Queue out"=w2744:refnum<queue>)  [unwired: 6 in]
        }
        n1189 = Merge Errors(w2711) -> (w2710:errorcluster)
        n1190 = Initialize Array(TRUE, 6 ("dimension size")) -> (w2688:bool[])
        n1191 = To Variant(anything=T3."mux10_1_channel4" ("mux10_1(x6)_encode")) -> (Variant=w2697:variant)
        n1192 = To Variant(anything=T4."demux1_10_channel4" ("demux1_10(x6)_encode")) -> (Variant=w2693:variant)
        n1193 = To Variant(anything=w2688) -> (Variant=w2687:variant)
        n1194 = Bundle By Name(cluster=w2685, "command"="MEAS.mux10-1", "data"=w2697) -> (w2692:T9)
        n1195 = Bundle By Name(cluster=w2685, "command"="MEAS.demux1-10", "data"=w2693) -> (w2691:T9)
        n1196 = Bundle By Name(cluster=w2685, "command"="MEAS.eMIC", "data"=w2687) -> (w2686:T9)
        n1197 = Build Array(w2692, w2691, w2686) -> (w2709:T9[])
        n1198 = Reverse 1D Array(array=w2709) -> (reversed array=w2708:T9[])
        n1199 = for {
          tunnel: w2708 -> [w2757] mode=indexing
          tunnel: [w2754] -> w2717 mode=indexing
          tunnel: w2710 -> [w2753]
          tunnel: w2713 -> [w2758]
          n1200 = Unbundle By Name(w2757) -> ("command"=w2756:string, "data"=w2755:variant)
          n1201 = call "App enquece.vi"("Priority Enquece"=TRUE, "error in (no error)"=w2753, "command data"=w2755, "command"=w2756, "queue in"=w2758) -> ("error out"=w2754:errorcluster)  [unwired: 5 in, 1 out]
        }
        n1202 = Merge Errors(w2720, w2717) -> (w2721:errorcluster)
      }
      frame "Test Channel 5" {
        w2760 = T9 {"command"="", "data"=variant} ("element")
        w2798 = 5  # DUT channel (1-11)
        n1203 = disable-structure shown="LOGGING==TRUE" {
          disable-tunnel: w2793 -> [w2824 _]
          frame condition #0 (active) {
            n1204 = Empty String/Path?(string/path=w2824) -> (empty?=w2826:bool)
            n1205 = Select(t="Quece timeout", s=w2826, f=w2824) -> (s? t:f=w2823:string)
            n1206 = call "string log (SubVI).vi"("state Name"=w2823) -> ()  [unwired: 9 in, 2 out]
          }
          frame condition #1 {
          }
        }
        n1207 = Build Array("Apps.UI Update", "MEAS.AllRelaysOFF2", "Apps.WaitForEvent") -> (w2781:string[])
        n1208 = for {
          tunnel: [w2814] -> w2788 mode=indexing
          shift-right: [w2815] -> w2789
          shift-left: w2783 -> [w2813]
          tunnel: w2781 -> [w2812] mode=indexing
          n1209 = call "App enquece.vi"("Priority Enquece"=TRUE, "command"=w2812, "queue in"=w2813) -> ("error out"=w2814:errorcluster, "Queue out"=w2815:refnum<queue>)  [unwired: 7 in]
        }
        n1210 = call "FGV DRV stand.vi"() -> ("Sub-Test.DCV"=w2774:bool)  [unwired: 10 in, 1 out]
        n1211 = case shown="True" w2774 {
          tunnel: [w2801 w2811] -> w2790
          frame False {
            n1212 = Build Array("WaitFor", "MEAS.requestAC") -> (w2801:string[])
          }
          frame True {
            n1213 = Build Array("Test DRV 25", "Test DRV 26", "Test DRV 27", "Test DRV 28", "Test DRV 29", "Test DRV 30", "MEAS.requestAC") -> (w2811:string[])
          }
        }
        n1214 = Merge Errors(w2788) -> (w2780:errorcluster)
        n1215 = Reverse 1D Array(array=w2790) -> (reversed array=w2791:string[])
        n1216 = for {
          tunnel: w2791 -> [w2821] mode=indexing
          tunnel: [w2820] -> w2787 mode=indexing
          shift-right: [w2819] -> w2779
          shift-left: w2789 -> [w2822]
          tunnel: w2780 -> [w2818]
          n1217 = call "App enquece.vi"("Priority Enquece"=TRUE, "error in (no error)"=w2818, "command"=w2821, "queue in"=w2822) -> ("error out"=w2820:errorcluster, "Queue out"=w2819:refnum<queue>)  [unwired: 6 in]
        }
        n1218 = Merge Errors(w2787) -> (w2786:errorcluster)
        n1219 = Initialize Array(TRUE, 6 ("dimension size")) -> (w2763:bool[])
        n1220 = To Variant(anything=T3."mux10_1_channel5" ("mux10_1(x6)_encode")) -> (Variant=w2772:variant)
        n1221 = To Variant(anything=T4."demux1_10_channel5" ("demux1_10(x6)_encode")) -> (Variant=w2768:variant)
        n1222 = To Variant(anything=w2763) -> (Variant=w2762:variant)
        n1223 = Bundle By Name(cluster=w2760, "command"="MEAS.mux10-1", "data"=w2772) -> (w2767:T9)
        n1224 = Bundle By Name(cluster=w2760, "command"="MEAS.demux1-10", "data"=w2768) -> (w2766:T9)
        n1225 = Bundle By Name(cluster=w2760, "command"="MEAS.eMIC", "data"=w2762) -> (w2761:T9)
        n1226 = Build Array(w2767, w2766, w2761) -> (w2785:T9[])
        n1227 = Reverse 1D Array(array=w2785) -> (reversed array=w2784:T9[])
        n1228 = for {
          tunnel: w2784 -> [w2833] mode=indexing
          tunnel: [w2830] -> w2792 mode=indexing
          tunnel: w2786 -> [w2829]
          tunnel: w2779 -> [w2827]
          n1229 = Unbundle By Name(w2833) -> ("command"=w2832:string, "data"=w2831:variant)
          n1230 = call "App enquece.vi"("Priority Enquece"=TRUE, "error in (no error)"=w2829, "command data"=w2831, "command"=w2832, "queue in"=w2827) -> ("error out"=w2830:errorcluster)  [unwired: 5 in, 1 out]
        }
        n1231 = Merge Errors(w2795, w2792) -> (w2796:errorcluster)
      }
      frame "Test Channel 6" {
        w2835 = T9 {"command"="", "data"=variant} ("element")
        w2873 = 6  # DUT channel (1-10)
        n1232 = disable-structure shown="LOGGING==TRUE" {
          disable-tunnel: w2868 -> [w2899 _]
          frame condition #0 (active) {
            n1233 = Empty String/Path?(string/path=w2899) -> (empty?=w2901:bool)
            n1234 = Select(t="Quece timeout", s=w2901, f=w2899) -> (s? t:f=w2898:string)
            n1235 = call "string log (SubVI).vi"("state Name"=w2898) -> ()  [unwired: 9 in, 2 out]
          }
          frame condition #1 {
          }
        }
        n1236 = Build Array("Apps.UI Update", "MEAS.AllRelaysOFF2", "Apps.WaitForEvent") -> (w2855:string[])
        n1237 = for {
          tunnel: [w2889] -> w2862 mode=indexing
          shift-right: [w2890] -> w2864
          shift-left: w2857 -> [w2888]
          tunnel: w2855 -> [w2887] mode=indexing
          n1238 = call "App enquece.vi"("Priority Enquece"=TRUE, "command"=w2887, "queue in"=w2888) -> ("error out"=w2889:errorcluster, "Queue out"=w2890:refnum<queue>)  [unwired: 7 in]
        }
        n1239 = call "FGV DRV stand.vi"() -> ("Sub-Test.DCV"=w2849:bool)  [unwired: 10 in, 1 out]
        n1240 = Merge Errors(w2862) -> (w2854:errorcluster)
        n1241 = case shown="True" w2849 {
          tunnel: [w2876 w2886] -> w2865
          frame False {
            n1242 = Build Array("WaitFor", "MEAS.requestAC") -> (w2876:string[])
          }
          frame True {
            n1243 = Build Array("Test DRV 31", "Test DRV 32", "Test DRV 33", "Test DRV 34", "Test DRV 35", "Test DRV 36", "MEAS.requestAC") -> (w2886:string[])
          }
        }
        n1244 = Reverse 1D Array(array=w2865) -> (reversed array=w2866:string[])
        n1245 = for {
          tunnel: w2866 -> [w2896] mode=indexing
          tunnel: [w2895] -> w2861 mode=indexing
          shift-right: [w2894] -> w2863
          shift-left: w2864 -> [w2897]
          tunnel: w2854 -> [w2893]
          n1246 = call "App enquece.vi"("Priority Enquece"=TRUE, "error in (no error)"=w2893, "command"=w2896, "queue in"=w2897) -> ("error out"=w2895:errorcluster, "Queue out"=w2894:refnum<queue>)  [unwired: 6 in]
        }
        n1247 = Merge Errors(w2861) -> (w2860:errorcluster)
        n1248 = Initialize Array(TRUE, 6 ("dimension size")) -> (w2838:bool[])
        n1249 = To Variant(anything=T3."mux10_1_channel6" ("mux10_1(x6)_encode")) -> (Variant=w2847:variant)
        n1250 = To Variant(anything=T4."demux1_10_channel6" ("demux1_10(x6)_encode")) -> (Variant=w2843:variant)
        n1251 = To Variant(anything=w2838) -> (Variant=w2837:variant)
        n1252 = Bundle By Name(cluster=w2835, "command"="MEAS.mux10-1", "data"=w2847) -> (w2842:T9)
        n1253 = Bundle By Name(cluster=w2835, "command"="MEAS.demux1-10", "data"=w2843) -> (w2841:T9)
        n1254 = Bundle By Name(cluster=w2835, "command"="MEAS.eMIC", "data"=w2837) -> (w2836:T9)
        n1255 = Build Array(w2842, w2841, w2836) -> (w2859:T9[])
        n1256 = Reverse 1D Array(array=w2859) -> (reversed array=w2858:T9[])
        n1257 = for {
          tunnel: w2858 -> [w2907] mode=indexing
          tunnel: [w2904] -> w2867 mode=indexing
          tunnel: w2860 -> [w2903]
          tunnel: w2863 -> [w2908]
          n1258 = Unbundle By Name(w2907) -> ("command"=w2906:string, "data"=w2905:variant)
          n1259 = call "App enquece.vi"("Priority Enquece"=TRUE, "error in (no error)"=w2903, "command data"=w2905, "command"=w2906, "queue in"=w2908) -> ("error out"=w2904:errorcluster)  [unwired: 5 in, 1 out]
        }
        n1260 = Merge Errors(w2870, w2867) -> (w2871:errorcluster)
      }
      frame "Test Channel 7" {
        w2934 = 7  # DUT channel (1-11)
        n1261 = disable-structure shown="LOGGING==TRUE" {
          disable-tunnel: w2929 -> [w2988 _]
          frame condition #0 (active) {
            n1262 = Empty String/Path?(string/path=w2988) -> (empty?=w2990:bool)
            n1263 = Select(t="Quece timeout", s=w2990, f=w2988) -> (s? t:f=w2987:string)
            n1264 = call "string log (SubVI).vi"("state Name"=w2987) -> ()  [unwired: 9 in, 2 out]
          }
          frame condition #1 {
          }
        }
